vi "for1.vi"() -> ()   [LabVIEW 2017]
panel:
  out "数组":dbl[][](array[numeric])
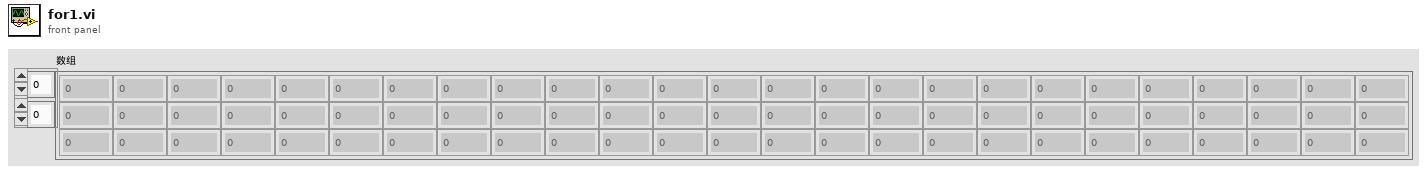
[diagram p1: front panel]
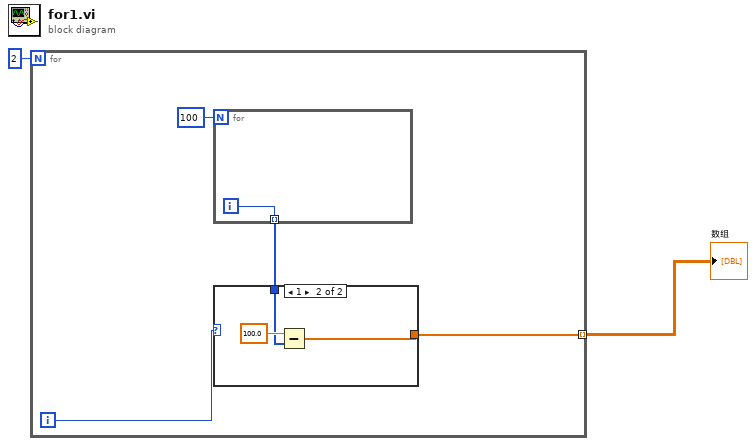
[diagram p0: block diagram]
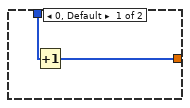
[diagram p2: hidden frame]
diagram:
  n1 = for {
    N: 2 -> [_]
    tunnel: [w3] -> w1 mode=indexing
    i -> [w5]
    n2 = for {
      N: 100 -> [_]
      tunnel: [w12] -> w4 mode=indexing
      i -> [w12]
    }
    n3 = case shown="1" w5 {
      tunnel: w4 -> [w8 w10]
      tunnel: [w7 w9] -> w3
      frame 0, Default {
        n4 = Increment(x=w8) -> (x+1=w7:i32[])
      }
      frame 1 {
        n5 = Subtract(x=100.0, y=w10) -> (x-y=w9:dbl[])
      }
    }
  }
  "数组" <- w1
